vi "RecordTipMovement (SubVi).vi"(6 "Pixel":i32=10000 min=1024 max=200000, 7 "time":sgl, 8 "error in (no error)":errorcluster, 9 "Y (m)":sgl min=-0.001 max=0.001 format="%.3p", 10 "X (m)":sgl min=-0.001 max=0.001 format="%.3p", 11 "Application ref in":refnum<vi>) -> (0 "error out":errorcluster, 1 "Data":sgl[][](array[numeric]), 2 "Channels indexes (0-23)":i32[](array[numeric]), 3 "Application ref out":refnum<vi>)   [LabVIEW 2014]
uses:
  <userlib>/Nanonis Prog Interface V5/Nanonis Prog Interface.lvlib
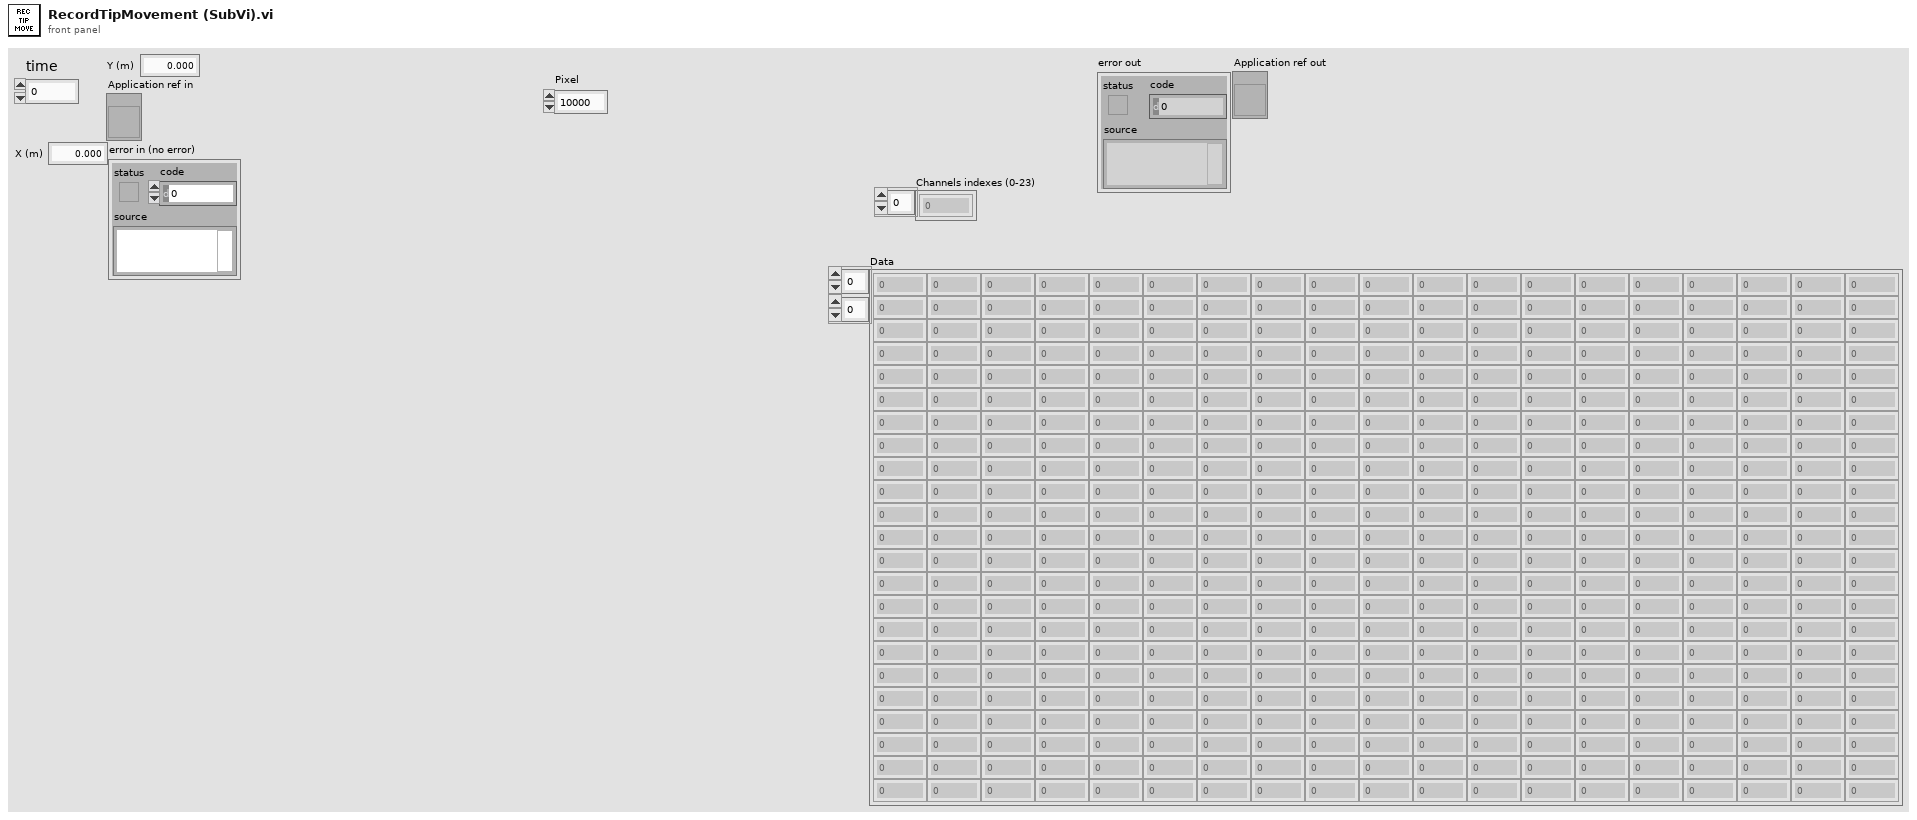
[diagram p1: front panel]
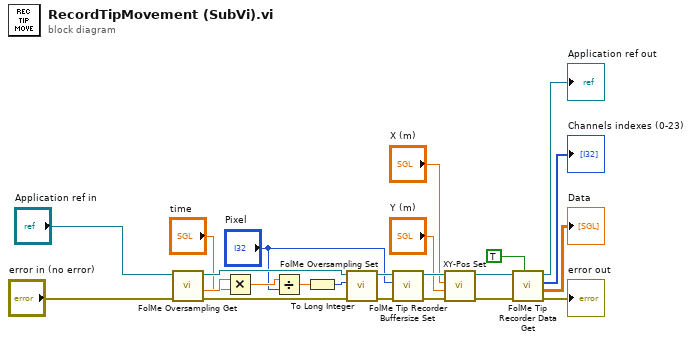
[diagram p0: block diagram]
diagram:
  n1 = call <userlib>:"FolMe Oversampling Get.vi"("error in (no error)"="error in (no error)", "Application ref in"="Application ref in") -> ("error out"=w10:errorcluster, "Sampling rate (S/s)"=w8:sgl, "Application ref out"=w9:refnum<vi>)  [unwired: 4 in, 1 out]
  n2 = Multiply(x=w8, y="time") -> (x*y=w7:sgl)
  n3 = Divide(x=w7, y="Pixel") -> (x/y=w5:sgl)
  n4 = To Long Integer(number=w5) -> (32bit integer=w4:i32)
  n5 = call <userlib>:"FolMe Oversampling Set.vi"("error in (no error)"=w10, "Oversampling"=w4, "Application ref in"=w9) -> ("error out"=w18:errorcluster, "Application ref out"=w20:refnum<vi>)  [unwired: 5 in]
  n6 = call <userlib>:"FolMe Tip Recorder Buffersize Set.vi"("error in (no error)"=w18, "Buffer size"="Pixel", "Application ref in"=w20) -> ("error out"=w14:errorcluster, "Application ref out"=w19:refnum<vi>)  [unwired: 5 in]
  n7 = call <userlib>:"XY-Pos Set.vi"("error in (no error)"=w14, "Y (m)"="Y (m)", "X (m)"="X (m)", "Application ref in"=w19) -> ("error out"=w13:errorcluster, "Application ref out"=w23:refnum<vi>)  [unwired: 4 in]
  n8 = call <userlib>:"FolMe Tip Recorder Data Get.vi"("Clear buffer? (F=False)"=TRUE ("Clear buffer? (False)"), "error in (no error)"=w13, "Application ref in"=w23) -> ("error out"=→"error out":errorcluster, "Data"=→"Data":sgl[][], "Channels indexes (0-23)"=→"Channels indexes (0-23)":i32[], "Application ref out"=→"Application ref out":refnum<vi>)  [unwired: 5 in]
